vi "tsapp_configure_baudrate_can_win32.vi"(1 "AppName":string, 2 "配置波特率":T1={"ABaudrateKbps"=0.0, "AListenOnly"=enum."Normal", "Int120Ohm"=enum."Disable", "EnableChannel"=enum."Disable", "AAppChannel"=0, "硬件类型"=8, "AHwChannel"=0} {"AHwChannel" items=["CHN1", "CHN2", "CHN3", "CHN4", "CHN5", "CHN6", "CHN7", "CHN8", "CHN9", "CHN10", "CHN11", "CHN12", "CHN13", "CHN14", "CHN15", "CHN16", "CHN17", "CHN18", "CHN19", "CHN20", "CHN21", "CHN22", "CHN23", "CHN24", "CHN25", "CHN26", "CHN27", "CHN28", "CHN29", "CHN30", "CHN31", "CHN32"]; "硬件类型" items=["BUS_UNKNOWN_TYPE", "TS_TCP_DEVICE", "XL_USB_DEVICE", "TS_USB_DEVICE", "PEAK_USB_DEVICE", "KVASER_USB_DEVICE", "ZLG_USB_DEVICE", "ICS_USB_DEVICE", "TS_TC1005_DEVICE"]; "AAppChannel" items=["CHN1", "CHN2", "CHN3", "CHN4", "CHN5", "CHN6", "CHN7", "CHN8", "CHN9", "CHN10", "CHN11", "CHN12", "CHN13", "CHN14", "CHN15", "CHN16", "CHN17", "CHN18", "CHN19", "CHN20", "CHN21", "CHN22", "CHN23", "CHN24", "CHN25", "CHN26", "CHN27", "CHN28", "CHN29", "CHN30", "CHN31", "CHN32"]}, 3 "错误输入（无错误）":errorcluster) -> (9 "InitSts":bool, 10 "错误输出":errorcluster)   [LabVIEW 2016]
uses:
  CAN_BaudInfo.ctl
  TSMaster.dll
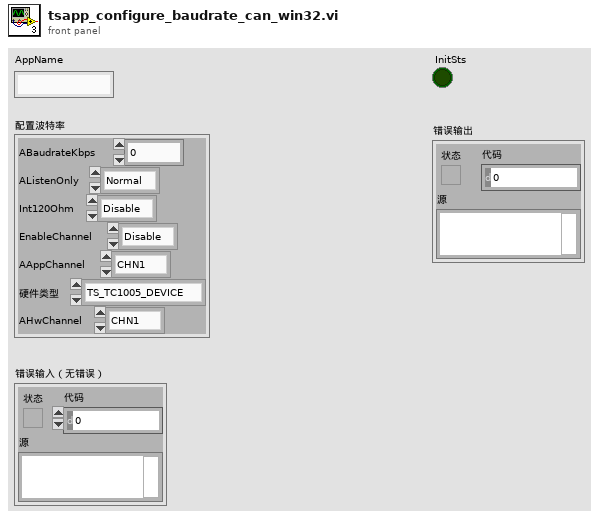
[diagram p1: front panel]
types:
  T1 = typedef "CAN_BaudInfo.ctl" = cluster{"ABaudrateKbps":sgl, "AListenOnly":enum16{"Normal", "ListenOnly"}, "Int120Ohm":enum16{"Disable", "Enable"}, "EnableChannel":enum16{"Disable", "Enable"}, "AAppChannel":i32, "硬件类型":i32, "AHwChannel":i32}
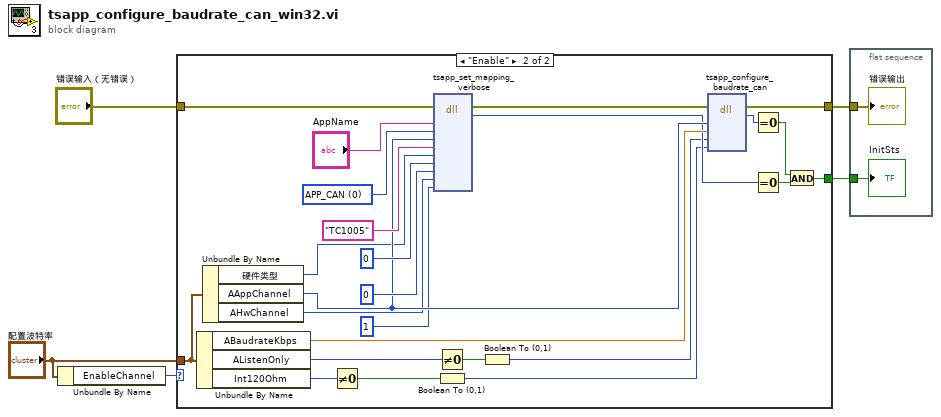
[diagram p0: block diagram]
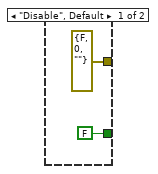
[diagram p2: hidden frame]
diagram:
  n1 = Unbundle By Name("配置波特率") -> ("EnableChannel"=w2:enum16{"Disable", "Enable"})
  n2 = case shown="\"Enable\"" w2 {
    tunnel: "错误输入（无错误）" -> [_ w31]
    tunnel: [errorcluster {"status"=FALSE, "code"=0, "source"=""} ("错误输出") w26] -> w4
    tunnel: [FALSE w12] -> w3
    tunnel: "配置波特率" -> [_ w19]
    frame "Disable", Default {
    }
    frame "Enable" {
      w30 = 0 items=["APP_CAN", "APP_LIN"] ("AAppChannelType")
      n3 = Unbundle By Name(w19) -> ("ABaudrateKbps"=w25:sgl, "AListenOnly"=w23:enum16{"Normal", "ListenOnly"}, "Int120Ohm"=w24:enum16{"Disable", "Enable"})
      n4 = Unbundle By Name(w19) -> ("硬件类型"=w11:i32, "AAppChannel"=w18:i32, "AHwChannel"=w17:i32)
      n5 = Not Equal To 0?(x=w24) -> (x != 0?=w21:bool)
      n6 = dll-call lib="C:/Users/Eric/Desktop/TSCAN_LV2010/TSMaster.dll" fn="tsapp_set_mapping_verbose"(error in=w31, "FAppName"="AppName", "AChnType"=w30, "FAppChannelIndex"=w18, "AHWDeviceName"="TC1005" ("AHardwareName"), "AHWDeviceType"=w11, "AHWDeviceSubType"=0 ("AHardwareIndex"), "AIdxHW"=0 ("AHardwareSubType"), "AIdxHWChn"=w17, "FMappingDisabled"=u32 1) -> (error out=w32:errorcluster, "tsapp_set_channel_mapping"=w15:i32)  [unwired: 11 in, 1 out]
      n7 = Not Equal To 0?(x=w23) -> (x != 0?=w22:bool)
      n8 = Boolean To (0,1)(Boolean=w21) -> (0, 1=w8:i16)
      n9 = Boolean To (0,1)(Boolean=w22) -> (0, 1=w9:i16)
      n10 = dll-call lib="C:/Users/Eric/Desktop/TSCAN_LV2010/TSMaster.dll" fn="tsapp_configure_baudrate_can"(error in=w32, "AIdxChn"=w18, "ABaudrateKbps"=w25, "AListenOnly"=w9, "AInstallTermResistor120Ohm"=w8) -> (error out=w26:errorcluster, "tsapp_configure_baudrate_can"=w16:i32)  [unwired: 6 in, 1 out]
      n11 = Equal To 0?(x=w16) -> (x = 0?=w14:bool)
      n12 = Equal To 0?(x=w15) -> (x = 0?=w13:bool)
      n13 = And(x=w14, y=w13) -> (x .and. y?=w12:bool)
    }
  }
  n14 = flat-sequence {
    tunnel: w4 -> [w34]
    tunnel: w3 -> [w33]
    frame #0 {
      "错误输出" <- w34
      "InitSts" <- w33
    }
  }
